vi "Config Setpoints.vi"(1 "Data In":T1) -> (0 "Data Out":T1)   [LabVIEW 2020]
uses:
  controls/UI Data.ctl
  controls/Setpoints.ctl
panel:
  in  "Disturbance pump 2":dbl caption="Amplitude"
  in  "Disturbance pump 1":dbl caption="Amplitude"
  in  "OK":bool caption="Blank"
  in  "Phase Tank2":dbl caption="Phase"
  in  "Frequency Tank2":dbl caption="Frequency"
  in  "Amplitude Tank2":dbl caption="Amplitude"
  in  "Phase Tank1":dbl caption="Phase"
  in  "Frequency Tank1":dbl caption="Frequency"
  in  "Amplitude Tank1":dbl caption="Amplitude"
  in  "Sin on-off":enum32{"On", "Off"}(radio)=enum."Off" caption="Radio Buttons"
  in  "Setpoint Tank 2":dbl(slide)=7.5 caption="Vertical Slider" scale=0.0..10.0 scale format="%#2_2g"
  in  "Setpoint Tank 1":dbl(slide)=7.5 caption="Vertical Slider" scale=0.0..10.0 scale format="%#2_2g"
  # "Sinusoidal Setpoints"
  # "Disturbance"
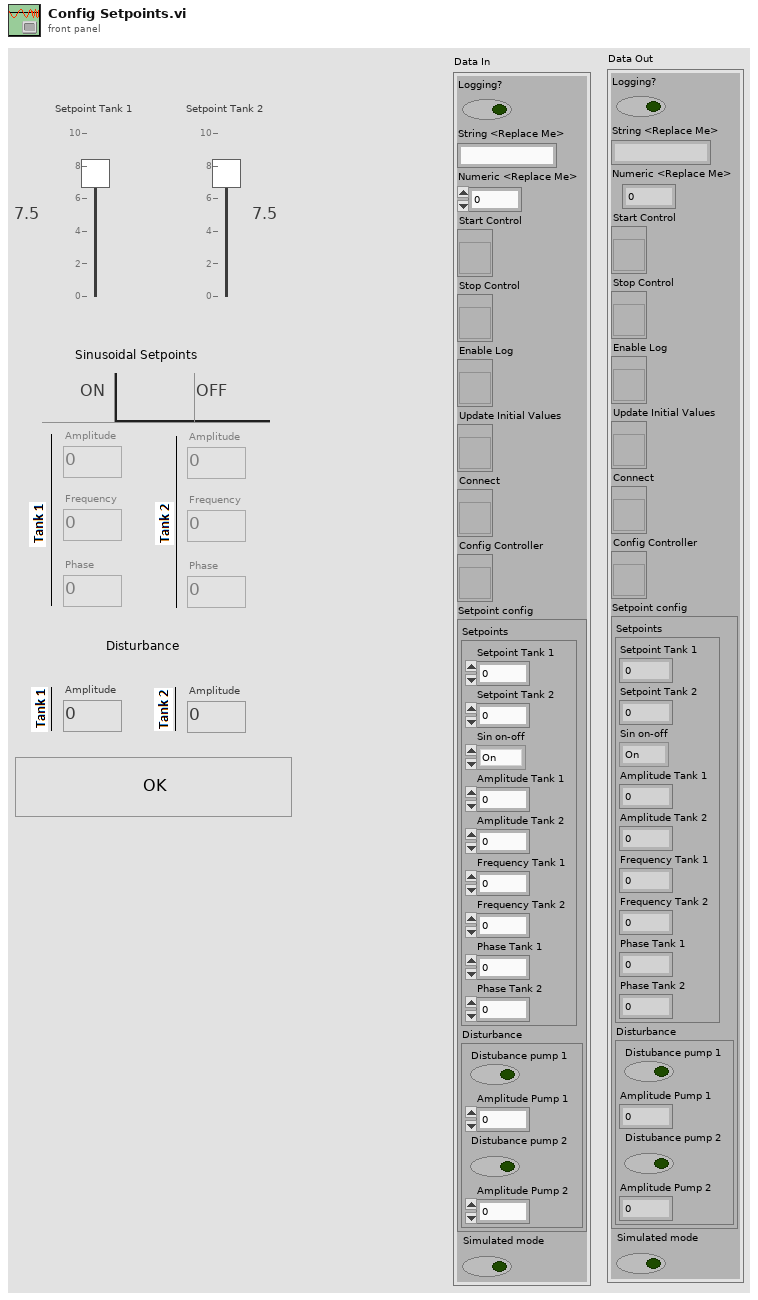
[diagram p1: front panel]
types:
  T1 = typedef "UI Data.ctl" = cluster{"Logging?":bool, "String <Replace Me>":string, "Numeric <Replace Me>":dbl, "Start Control":refnum<vi>, "Stop Control":refnum<vi>, "Enable Log":refnum<vi>, "Update Initial Values":refnum<vi>, "Connect":refnum<vi>, "Config Controller":refnum<vi>, "Setpoint config":T2, "Simulated mode":bool}
  T2 = typedef "Setpoints.ctl" = cluster{"Setpoints":cluster{"Setpoint Tank 1":dbl, "Setpoint Tank 2":dbl, "Sin on-off":enum32{"On", "Off"}, "Amplitude Tank 1":dbl, "Amplitude Tank 2":dbl, "Frequency Tank 1":dbl, "Frequency Tank 2":dbl, "Phase Tank 1":dbl, "Phase Tank 2":dbl}, "Disturbance":cluster{"Distubance pump 1":bool, "Amplitude Pump 1":dbl, "Distubance pump 2":bool, "Amplitude Pump 2":dbl}}
  T3 = enum8{"Enabled", "Disabled", "Disabled and Grayed Out"}
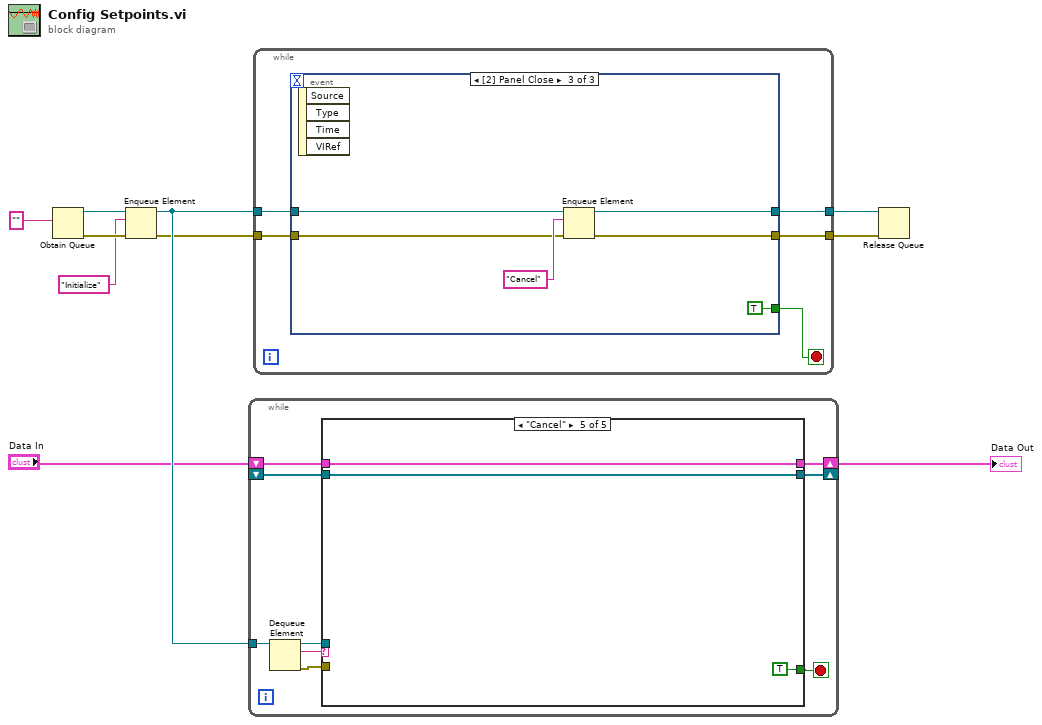
[diagram p0: block diagram]
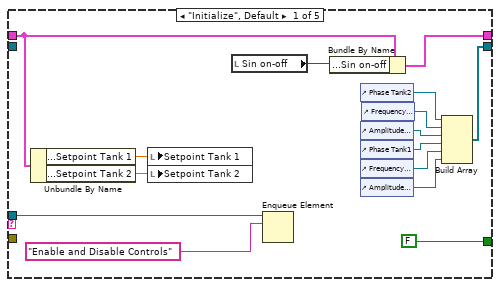
[diagram p2: hidden frame]
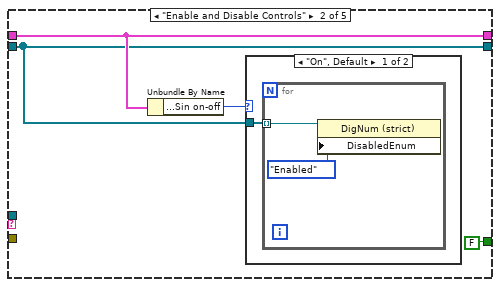
[diagram p3: hidden frame]
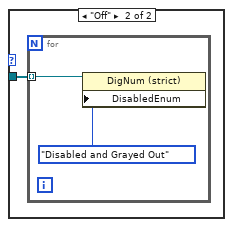
[diagram p4: hidden frame]
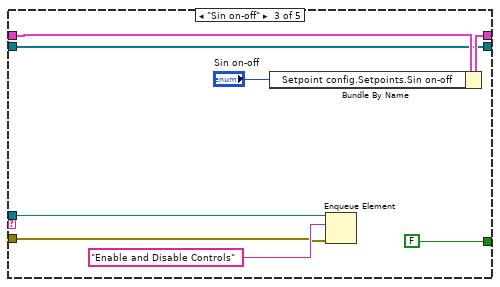
[diagram p5: hidden frame]
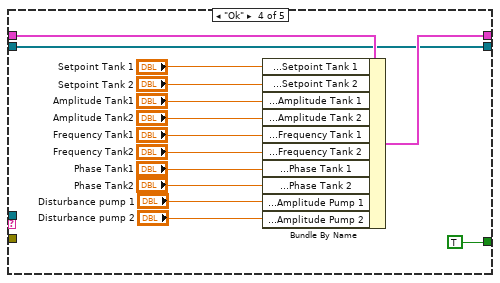
[diagram p6: hidden frame]
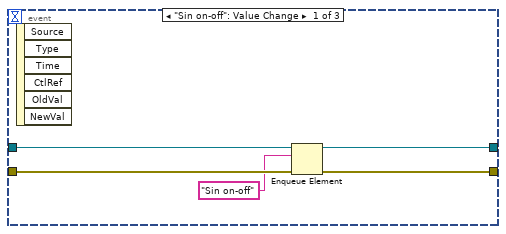
[diagram p7: hidden frame]
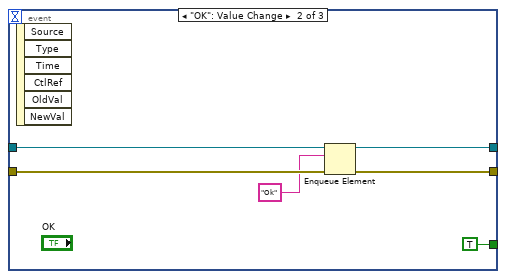
[diagram p8: hidden frame]
diagram:
  n1 = Obtain Queue(element data type="" ("element")) -> (queue out=w8:refnum<queue>, error out=w6:errorcluster)  [unwired: 4 in, 1 out]
  n2 = Enqueue Element(queue=w8, element="Initialize", error in (no error)=w6) -> (queue out=w7:refnum<queue>, error out=w5:errorcluster)  [unwired: 1 in, 1 out]
  n3 = while {
    tunnel: w7 -> [w19]
    shift-right: [w14] -> w1
    shift-left: "Data In" -> [w15]
    shift-right: [w12] -> _
    shift-left: _ -> [w11]
    stop <- w16 stop-if-true
    n4 = Dequeue Element(queue=w19) -> (queue out=w17:refnum<queue>, element=w18:string, error out=w13:errorcluster)  [unwired: 2 in, 1 out]
    n5 = case shown="\"Cancel\"" w18 {
      tunnel: w17 -> [w34 _ w47 _ _]
      tunnel: [FALSE FALSE FALSE TRUE TRUE] -> w16
      tunnel: w15 -> [w22 w38 w50 w65 w69]
      tunnel: [w31 w38 w49 w56 w69] -> w14
      tunnel: w13 -> [_ _ w46 _ _]
      tunnel: [w23 w35 w45 w53 w68] -> w12
      tunnel: w11 -> [_ w35 w45 w53 w68]
      frame "Initialize", Default {
        n6 = Unbundle By Name(w22) -> ("Setpoint config.Setpoints.Setpoint Tank 1"=w21:dbl, "Setpoint config.Setpoints.Setpoint Tank 2"=w20:dbl)
        n7 = local write "Setpoint Tank 1"(w21) -> ()
        n8 = local write "Setpoint Tank 2"(w20) -> ()
        n9 = local read "Sin on-off"() -> (w30:enum32{"On", "Off"})
        n10 = Enqueue Element(queue=w34, element="Enable and Disable Controls") -> ()  [unwired: 2 in, 3 out]
        n11 = Bundle By Name(cluster=w22, "Setpoint config.Setpoints.Sin on-off"=w30) -> (w31:T1)
        n12 = control-ref of="Phase Tank2"() -> (w24:refnum<vi>)
        n13 = control-ref of="Amplitude Tank2"() -> (w26:refnum<vi>)
        n14 = control-ref of="Phase Tank1"() -> (w29:refnum<vi>)
        n15 = control-ref of="Frequency Tank1"() -> (w27:refnum<vi>)
        n16 = control-ref of="Amplitude Tank1"() -> (w28:refnum<vi>)
        n17 = control-ref of="Frequency Tank2"() -> (w25:refnum<vi>)
        n18 = Build Array(w24, w25, w26, w29, w27, w28) -> (w23:refnum<vi>[])
      }
      frame "Enable and Disable Controls" {
        n19 = Unbundle By Name(w38) -> ("Setpoint config.Setpoints.Sin on-off"=w36:enum32{"On", "Off"})
        n20 = case shown="\"On\", Default" w36 {
          tunnel: w35 -> [w39 w42]
          frame "On", Default {
            n21 = for {
              tunnel: w39 -> [w40] mode=indexing
              n22 = property class="DigNum (strict)"(reference=w40, "DisabledEnum"=T3."Enabled" ("Disabled")) -> ()  [unwired: 1 in, 2 out]
            }
          }
          frame "Off" {
            n23 = for {
              tunnel: w42 -> [w43] mode=indexing
              n24 = property class="DigNum (strict)"(reference=w43, "DisabledEnum"=T3."Disabled and Grayed Out" ("Disabled")) -> ()  [unwired: 1 in, 2 out]
            }
          }
        }
      }
      frame "Sin on-off" {
        n25 = Bundle By Name(cluster=w50, "Setpoint config.Setpoints.Sin on-off"="Sin on-off") -> (w49:T1)
        n26 = Enqueue Element(queue=w47, element="Enable and Disable Controls", error in (no error)=w46) -> ()  [unwired: 1 in, 3 out]
      }
      frame "Ok" {
        n27 = Bundle By Name(cluster=w65, "Setpoint config.Setpoints.Setpoint Tank 1"="Setpoint Tank 1", "Setpoint config.Setpoints.Setpoint Tank 2"="Setpoint Tank 2", "Setpoint config.Setpoints.Amplitude Tank 1"="Amplitude Tank1", "Setpoint config.Setpoints.Amplitude Tank 2"="Amplitude Tank2", "Setpoint config.Setpoints.Frequency Tank 1"="Frequency Tank1", "Setpoint config.Setpoints.Frequency Tank 2"="Frequency Tank2", "Setpoint config.Setpoints.Phase Tank 1"="Phase Tank1", "Setpoint config.Setpoints.Phase Tank 2"="Phase Tank2", "Setpoint config.Disturbance.Amplitude Pump 1"="Disturbance pump 1", "Setpoint config.Disturbance.Amplitude Pump 2"="Disturbance pump 2") -> (w56:T1)
      }
      frame "Cancel" {
      }
    }
  }
  "Data Out" <- w1
  n28 = while {
    tunnel: w7 -> [w74]
    tunnel: [w73] -> w10
    tunnel: w5 -> [w72]
    tunnel: [w71] -> w9
    stop <- w70 stop-if-true
    n29 = event shown="[2] Panel Close" {
      selector: _ -> [_ _ _]
      dyn-events: _ -> [_ _ _]
      timeout: _ -> [_ _ _]
      tunnel: w74 -> [w79 w85 w90]
      tunnel: [w78 w84 w87] -> w73
      tunnel: w72 -> [w77 w83 w89]
      tunnel: [w76 w82 w88] -> w71
      tunnel: [_ TRUE TRUE] -> w70
      event "Sin on-off": Value Change {
        n30 = event-data() -> ()  [unwired: 1 in, 6 out]
        n31 = Enqueue Element(queue=w79, element="Sin on-off", error in (no error)=w77) -> (queue out=w78:refnum<queue>, error out=w76:errorcluster)  [unwired: 1 in, 1 out]
      }
      event "OK": Value Change {
        n32 = event-data() -> ()  [unwired: 1 in, 6 out]
        n33 = Enqueue Element(queue=w85, element="Ok", error in (no error)=w83) -> (queue out=w84:refnum<queue>, error out=w82:errorcluster)  [unwired: 1 in, 1 out]
      }
      event Panel Close {
        n34 = event-data() -> ()  [unwired: 1 in, 4 out]
        n35 = Enqueue Element(queue=w90, element="Cancel", error in (no error)=w89) -> (queue out=w87:refnum<queue>, error out=w88:errorcluster)  [unwired: 1 in, 1 out]
      }
    }
  }
  n36 = Release Queue(queue=w10, error in (no error)=w9) -> ()  [unwired: 1 in, 3 out]
